vi "initialize Session Data.vi"(0 "Session in":refnum<class "SmartScopeDriver.lvclass">, 11 "error in":errorcluster) -> (4 "Session out":refnum<class "SmartScopeDriver.lvclass">, 15 "error out":errorcluster)   [LabVIEW 2019, in "SmartScopeDriver.lvclass"]
uses:
  SmartScopeDriver.lvclass
  <userlib>/_Session Fwk/Session - Root.lvclass
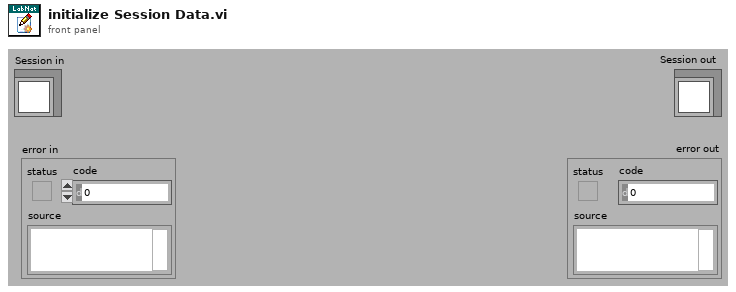
[diagram p1: front panel]
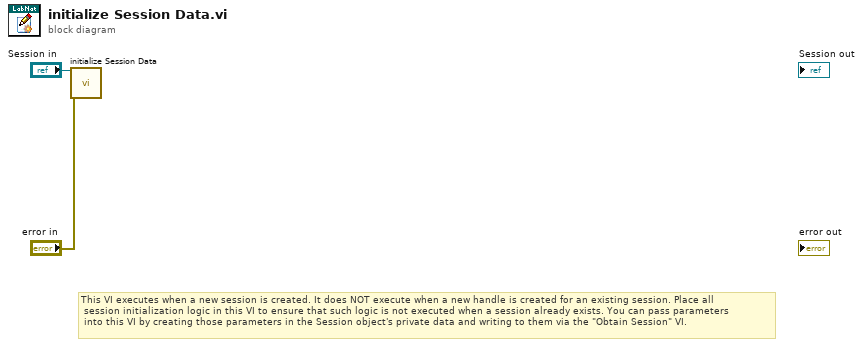
[diagram p0: block diagram]
diagram:
  # "This VI executes when a new session is created. It does NOT execute when a new handle is created for an existing session. Place all\n session initialization logic in this VI to ensure that such logic is not executed when a session already exists. You can pass parameters\n into this VI by creating those parameters in the Session object's private data and writing to them via the \"Obtain Session\" VI."
  n1 = call-parent "initialize Session Data.vi"("OBJ - Session in"="Session in", "error in"="error in") -> ("OBJ - Session out"=w3:refnum<class "SmartScopeDriver.lvclass">, "error out"=w1:errorcluster)  [unwired: 12 in]
